vi "PM100D Read.vi"() -> ()   [LabVIEW 2014]
doc: "This VI shows how to communicate with a PM100D optical power/energy meter with SCPI commands.\n- Initializing the instrument\n- Getting system info\n- Setting parameters\n- Measurement configuration\n- Measuring queue\n- Fetching and displaying a measurement value\n- Closing the application"
uses:
  Main-Stage-PI/(Global) Current handle and LaserPower_YCC.vi
  <vilib>/Utility/file.llb/Write To Spreadsheet File (DBL).vi
panel:
  in  "Save?":bool
  out "time had recorded (s)":dbl
  in  "Record time (s)":dbl
  out "Readout value (mW)":dbl format="%^#_9e"
  out "IDN String":string
  out "Sensor SN":string
  out "Sensor Name":string
  out "Sensor Flags":bool[](array[boolean])
  out "New":bool
  in  "Timeout [ms]":i32=1000
  in  "stop":bool
  in  "Readout Config":string(combo)="POW"
  out "Readout string":string
  out "Error log":string
  in  "Averaging Rate":i32=1
  # "1 Power Sensor"
  # "2 Energy Sensor"
  # "4"
  # "8"
  # "16 Response settable"
  # "32 Wavelength settable"
  # "64 Tau (time constant) settable"
  # "128"
  # "256 With temperature sensor"
  # "1000 mV= 7.378 mW"
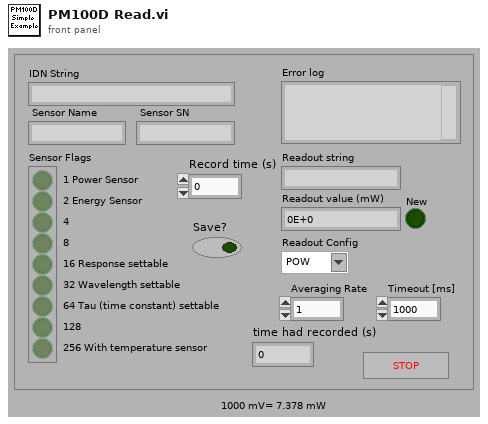
[diagram p1: front panel]
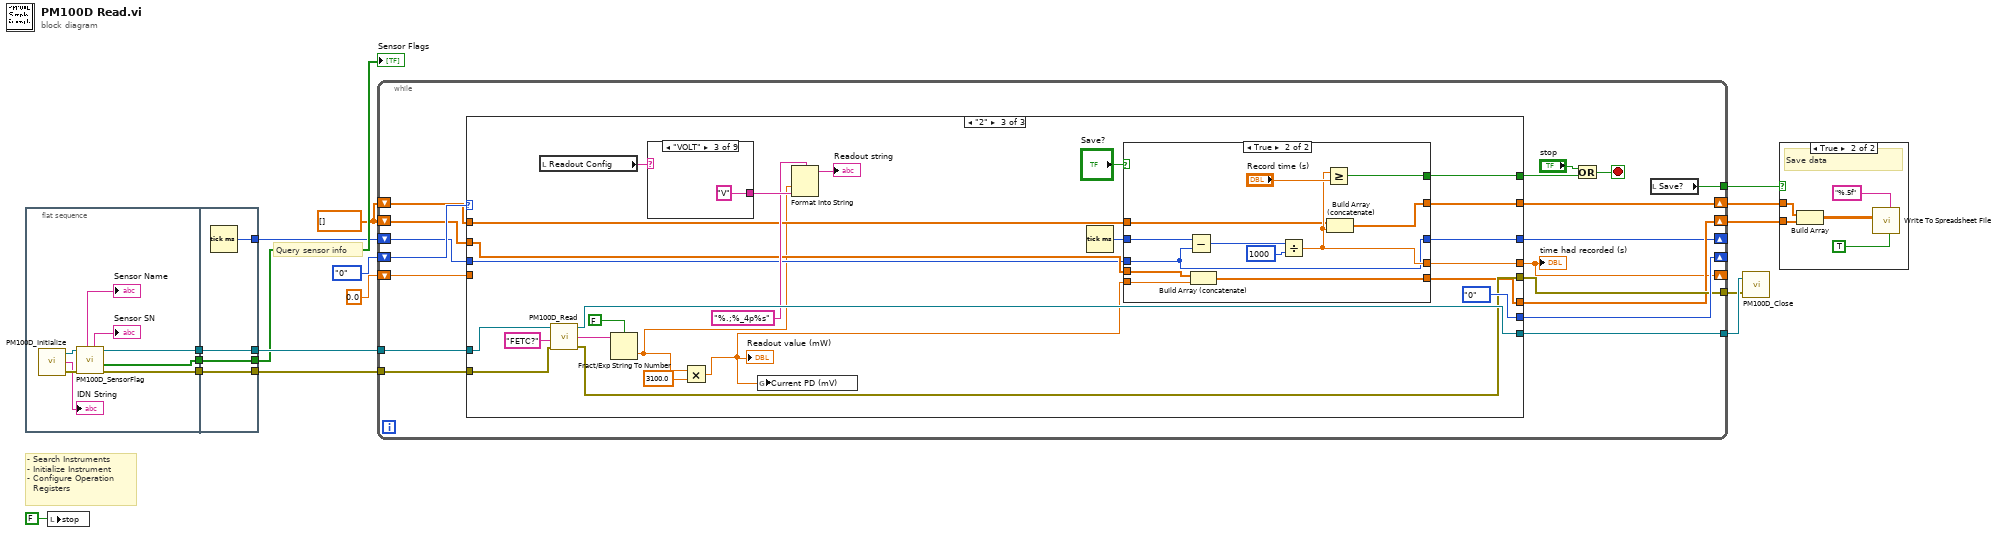
[diagram p0: block diagram]
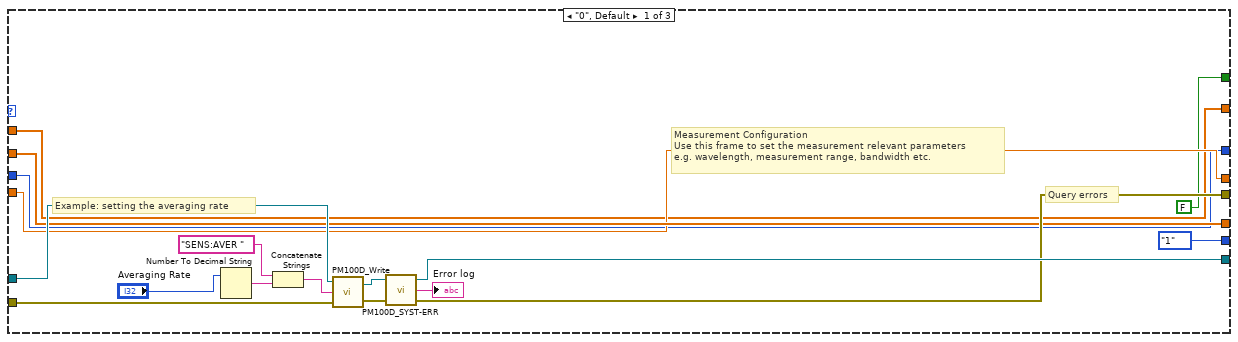
[diagram p3: hidden frame]
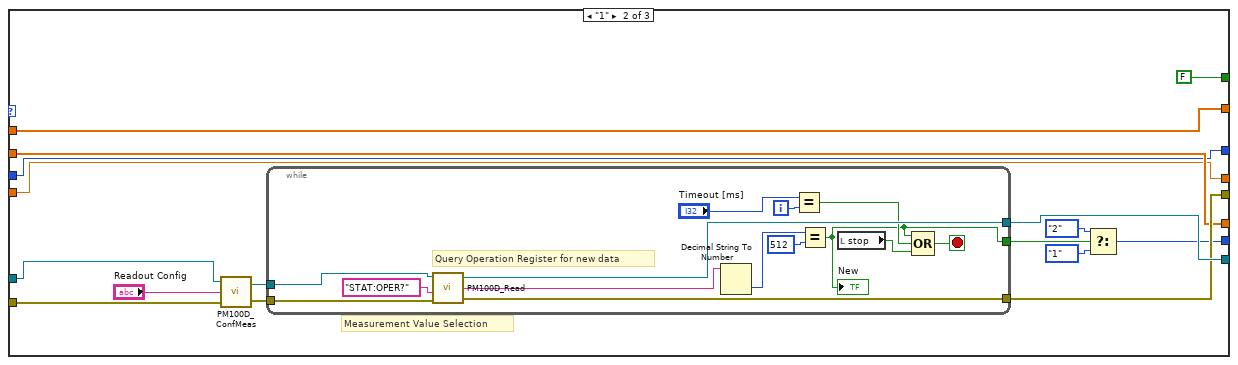
[diagram p4: hidden frame]
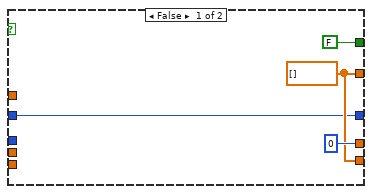
[diagram p5: hidden frame]
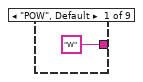
[diagram p6: hidden frame]
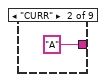
[diagram p7: hidden frame]
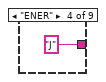
[diagram p8: hidden frame]
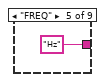
[diagram p9: hidden frame]
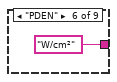
[diagram p10: hidden frame]
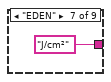
[diagram p11: hidden frame]
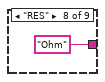
[diagram p12: hidden frame]
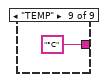
[diagram p13: hidden frame]
diagram:
  w5 = dbl[] []
  # "- Search Instruments\n- Initialize Instrument\n- Configure Operation\n  Registers"
  # "Query sensor info"
  n1 = flat-sequence {
    tunnel: [w22] -> w4
    tunnel: [w21] -> w3
    tunnel: [w20] -> w2
    tunnel: [w26] -> w14
    tunnel: [w27] -> w15
    tunnel: [w28] -> w16
    tunnel: w4 -> [w28]
    tunnel: w3 -> [w27]
    tunnel: w2 -> [w26]
    tunnel: [w25] -> w1
    frame #0 {
      n2 = call "PM100D_Initialize.vi"() -> ("error out"=w23:errorcluster, "Instrument"=→"IDN String":string, "VISA out"=w24:refnum<visa-resource-name>)  [unwired: 2 in, 1 out]
      n3 = call "PM100D_SensorFlag.vi"("error in (no error)"=w23, "VISA in"=w24) -> ("error out"=w21:errorcluster, "flags"=w20:bool[], "VISA out"=w22:refnum<visa-resource-name>, "sn"=→"Sensor SN":string, "name"=→"Sensor Name":string)  [unwired: 2 in, 3 out]
    }
    frame #1 {
      n4 = Tick Count (ms)() -> (millisecond timer value=w25:u32)
    }
  }
  n5 = local write "stop"(FALSE ("stop")) -> ()
  n6 = while {
    tunnel: w16 -> [w46]
    tunnel: w15 -> [w45]
    shift-right: [w43] -> _
    shift-left: enum16{"0", "1", "2"}."0" -> [w44]
    tunnel: [w42] -> w12
    tunnel: [w41] -> w11
    shift-right: [w37] -> w8
    shift-left: w5 -> [w38]
    shift-right: [w29] -> _
    shift-left: w1 -> [w36]
    tunnel: [w35] -> w9
    shift-right: [w33] -> _
    shift-left: 0.0 ("millisecond timer value") -> [w34]
    shift-right: [w32] -> w6
    shift-left: w5 -> [w31]
    stop <- w39 stop-if-true
    n7 = case shown="\"2\"" w44 {
      tunnel: w46 -> [w61 w79 w116]
      tunnel: w45 -> [w56 w78 w115]
      tunnel: [enum16{"0", "1", "2"}."1" w73 enum16{"0", "1", "2"}."0"] -> w43
      tunnel: [w54 w75 w114] -> w42
      tunnel: [w53 w74 w107] -> w41
      tunnel: w38 -> [w51 w68 w106]
      tunnel: [w51 w68 w105] -> w37
      tunnel: w36 -> [w47 w64 w104]
      tunnel: [w50 w67 w102] -> w33
      tunnel: w34 -> [w50 w67 _]
      tunnel: [w49 w66 w101] -> w32
      tunnel: w31 -> [w49 w66 w100]
      tunnel: [FALSE FALSE w99] -> w30
      tunnel: [w47 w64 w98] -> w29
      frame "0", Default {
        # "Query errors"
        # "Example: setting the averaging rate"
        # "Measurement Configuration\nUse this frame to set the measurement relevant parameters\ne.g. wavelength, measurement range, bandwidth etc."
        n8 = Number To Decimal String(number="Averaging Rate") -> (decimal integer string=w62:string)  [unwired: 1 in]
        n9 = Concatenate Strings("SENS:AVER " ("string"), w62) -> (w60:string)
        n10 = call "PM100D_Write.vi"("error in (no error)"=w56, "Command"=w60, "VISA in"=w61) -> ("error out"=w57:errorcluster, "VISA out"=w59:refnum<visa-resource-name>)
        n11 = call "PM100D_SYST-ERR.vi"("error out 2"=w57, "VISA In"=w59) -> ("error out"=w53:errorcluster, "Error"=→"Error log":string, "VISA Out"=w54:refnum<visa-resource-name>)  [unwired: 1 in]
      }
      frame "1" {
        # "Measurement Value Selection"
        n12 = call "PM100D_ConfMeas.vi"("error in"=w78, "Conf:"="Readout Config", "VISA In"=w79) -> ("error out"=w76:errorcluster, "dup VISA session"=w77:refnum<visa-resource-name>)
        n13 = while {
          tunnel: w77 -> [w89]
          tunnel: w76 -> [w88]
          tunnel: [w87] -> w75
          tunnel: [w86] -> w74
          tunnel: [w80] -> w70
          i -> [w82]
          stop <- w84 stop-if-true
          # "Query Operation Register for new data"
          n14 = call "PM100D_Read.vi"("error in (no error)"=w88, "Command"="STAT:OPER?", "VISA in"=w89) -> ("error out"=w86:errorcluster, "ReadValue"=w92:string, "VISA out"=w87:refnum<visa-resource-name>)  [unwired: 1 in]
          n15 = Decimal String To Number(string=w92) -> (number=w91:i32)  [unwired: 2 in, 1 out]
          n16 = Equal?(x="Timeout [ms]", y=w82) -> (x = y?=w81:bool)
          n17 = Equal?(x=w91, y=512) -> (x = y?=w80:bool)
          "New" <- w80
          n18 = local read "stop"() -> (w85:bool)
          n19 = Compound Arithmetic op=OR(w80, w81, w85) -> (w84:bool)
        }
        n20 = Select(t=enum16{"0", "1", "2"}."2", s=w70, f=enum16{"0", "1", "2"}."1") -> (s? t:f=w73:enum16{"0", "1", "2"})
      }
      frame "2" {
        n21 = local read "Readout Config"() -> (w113:string)
        n22 = call "PM100D_Read.vi"("error in (no error)"=w115, "Command"="FETC?", "VISA in"=w116) -> ("error out"=w107:errorcluster, "ReadValue"=w112:string, "VISA out"=w114:refnum<visa-resource-name>)  [unwired: 1 in]
        n23 = Fract/Exp String To Number(use system decimal point (T)=FALSE, string=w112) -> (number=w96:dbl)  [unwired: 2 in, 1 out]
        n24 = case shown="\"VOLT\"" w113 {
          tunnel: ["W" "A" "V" "J" "Hz" "W/cm²" "J/cm²" "Ohm" "°C"] -> w109
          frame "POW", Default {
          }
          frame "CURR" {
          }
          frame "VOLT" {
          }
          frame "ENER" {
          }
          frame "FREQ" {
          }
          frame "PDEN" {
          }
          frame "EDEN" {
          }
          frame "RES" {
          }
          frame "TEMP" {
          }
        }
        n25 = Multiply(x=w96, y=3100.0) -> (x*y=w94:dbl)
        "Readout value (mW)" <- w94
        n26 = global write "(Global) Current handle and LaserPower_YCC.vi" "Current PD (mV)"(w94) -> ()
        n27 = Format Into String(format string="%.;%_4p%s", w96, w109) -> (resulting string=→"Readout string":string)  [unwired: 2 in, 1 out]
        n28 = Tick Count (ms)() -> (millisecond timer value=w97:u32)
        n29 = case shown="True" "Save?" {
          tunnel: [u32 0 ("millisecond timer value") w127] -> w102
          tunnel: [FALSE w130] -> w99
          tunnel: w94 -> [_ w134]
          tunnel: [w120 w133] -> w105
          tunnel: w106 -> [_ w129]
          tunnel: w104 -> [_ w124]
          tunnel: [w120 w126] -> w101
          tunnel: w100 -> [_ w125]
          tunnel: [w119 w124] -> w98
          tunnel: w97 -> [w119 w123]
          frame False {
            w120 = dbl[] []
          }
          frame True {
            n30 = Subtract(x=w123, y=w124) -> (x-y=w128:u32)
            n31 = Build Array (concatenate)(w129, w134) -> (w133:dbl[])
            n32 = Divide(x=w128, y=1000) -> (x/y=w127:dbl)
            n33 = Greater Or Equal?(x=w127, y="Record time (s)") -> (x >= y?=w130:bool)
            n34 = Build Array (concatenate)(w125, w127) -> (w126:dbl[])
          }
        }
      }
    }
    "time had recorded (s)" <- w33
    n35 = Or(x="stop", y=w30) -> (x .or. y?=w39:bool)
    n36 = local read "Save?"() -> (w35:bool)
  }
  n37 = call "PM100D_Close.vi"("error in (no error)"=w11, "VISA resource name"=w12) -> ()  [unwired: 2 in]
  n38 = case shown="True" w9 {
    tunnel: w8 -> [_ w145]
    tunnel: w6 -> [_ w146]
    frame False {
    }
    frame True {
      # "Save data"
      n39 = Build Array(w146, w145) -> (w144:dbl[][])
      n40 = call-poly <vilib>:"Write To Spreadsheet File.vi"("transpose? (no:F)"=TRUE, "format (%.3f)"="%.5f", "2D data"=w144) -> ()  [unwired: 5 in, 1 out]
    }
  }
  "Sensor Flags" <- w14
